vi "Description.vi"(8 "error in (no error)":errorcluster, 11 "Comparator in":refnum<class "Comparator.lvclass">) -> (0 "error out":errorcluster, 2 "Description":string)   [LabVIEW 2020, in "Comparator.lvclass"]
uses:
  Comparator.lvclass
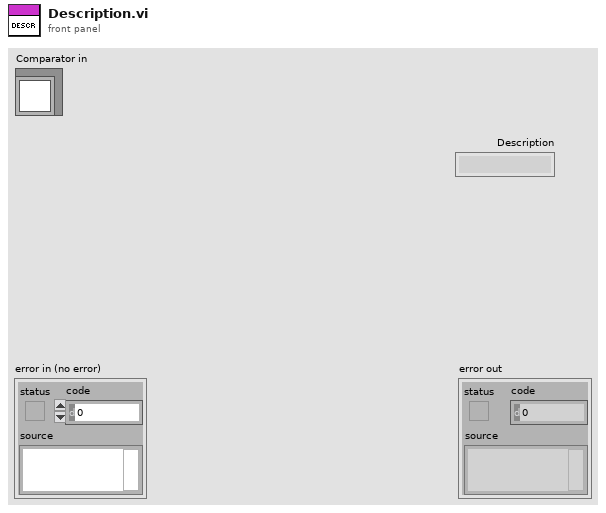
[diagram p1: front panel]
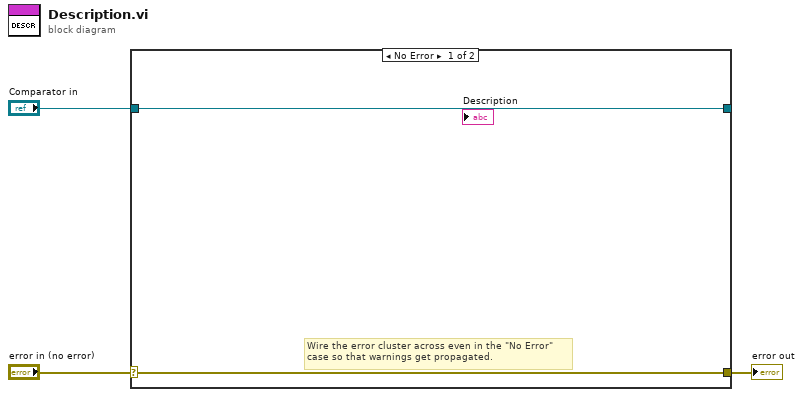
[diagram p0: block diagram]
diagram:
  n1 = case shown="No Error" "error in (no error)" {
    selector: "error in (no error)" -> [w4 w7]
    tunnel: [w4 w7] -> w2
    tunnel: [w5 w6] -> _
    tunnel: "Comparator in" -> [w5 w6]
    frame No Error {
      # "Wire the error cluster across even in the \"No Error\"\ncase so that warnings get propagated."
    }
    frame Error {
    }
  }
  "error out" <- w2
